vi "Modified Data File Current Mode_2.vi"(7 "Current Mode":u8[][](array[numeric]), 8 "modified error":errorcluster, 9 "modified data":path=path "C:/Users/User/Desktop/test.csv", 10 "original error":errorcluster, 11 "original data":path=path "C:/Users/User/Desktop/test.csv") -> (0 "modified data error out":errorcluster, 1 "modified data out":path, 2 "original error out":errorcluster, 3 "original data out":path)   [LabVIEW 2023]
uses:
  <vilib>/Utility/error.llb/DialogType.ctl
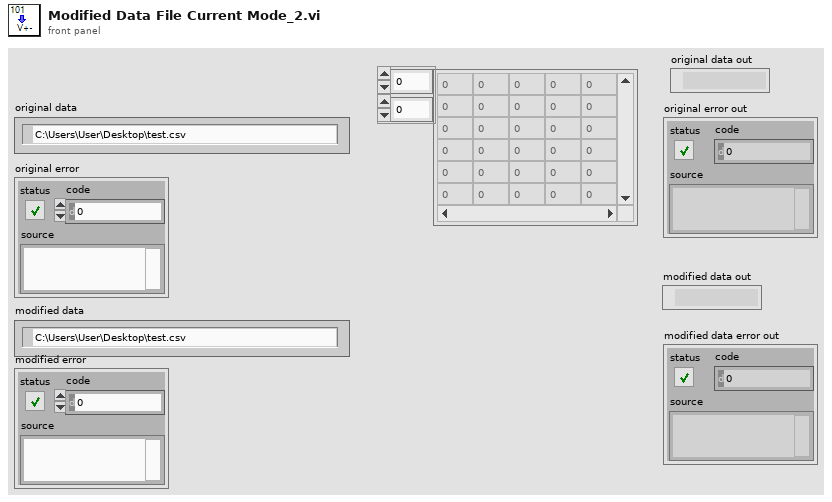
[diagram p1: front panel]
types:
  T1 = enum16{"open", "replace", "create", "open or create", "replace or create", "replace or create with confirmation"}
  T2 = typedef "DialogType.ctl" = u16
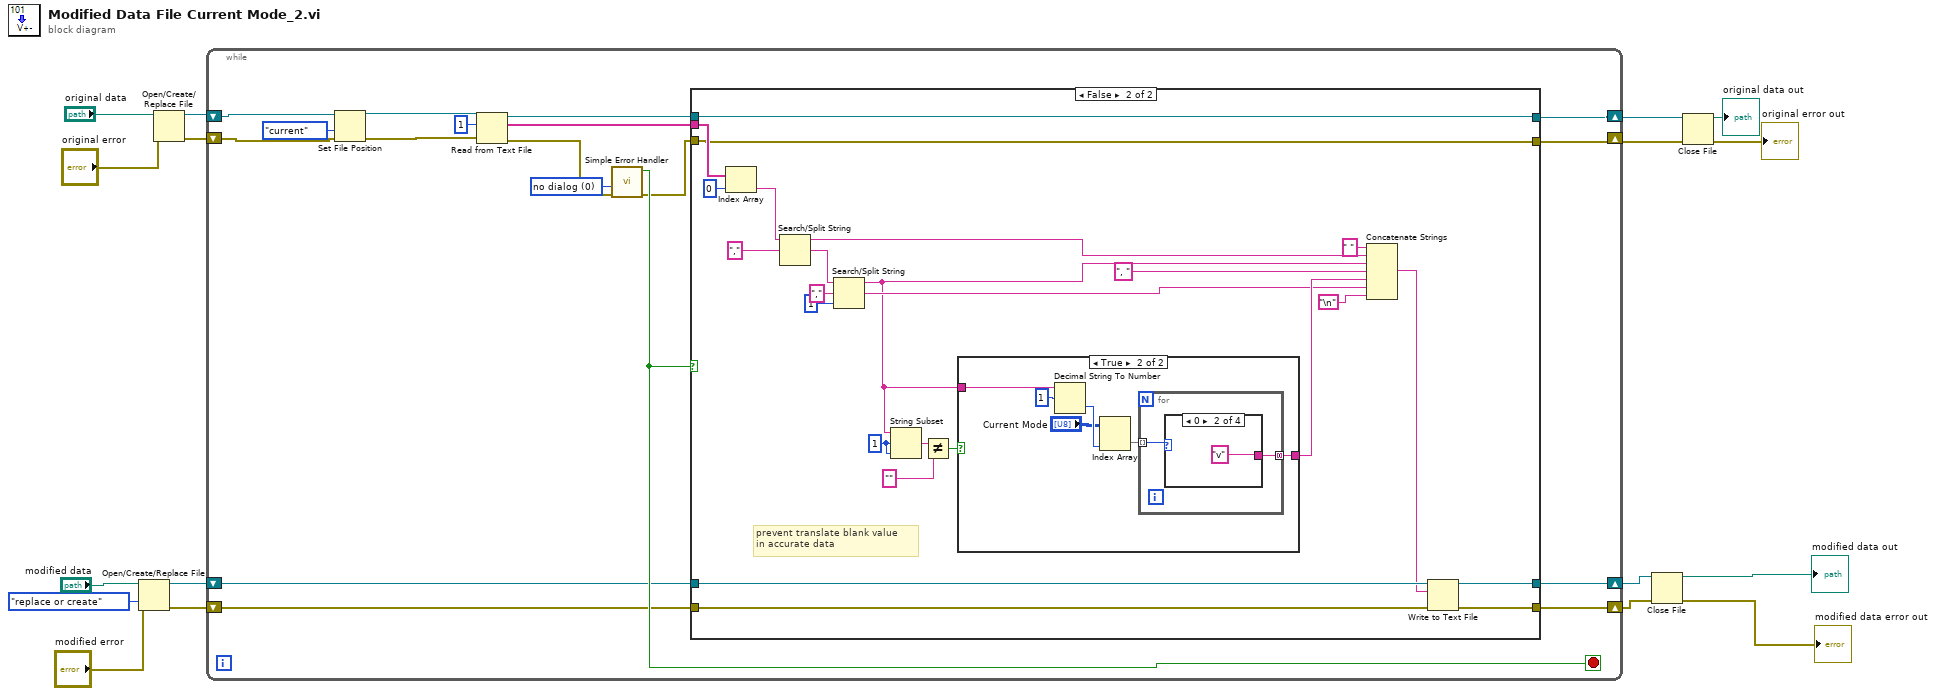
[diagram p0: block diagram]
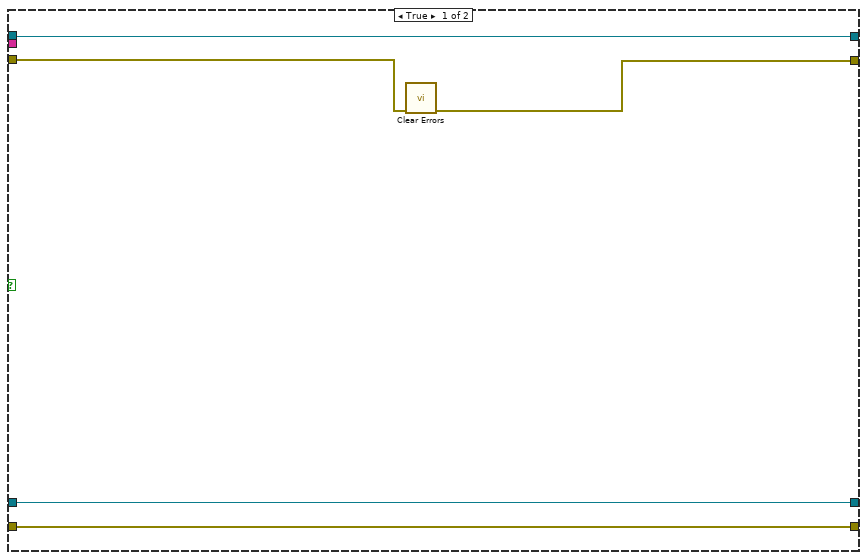
[diagram p2: hidden frame]
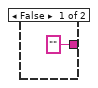
[diagram p3: hidden frame]
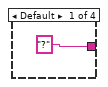
[diagram p4: hidden frame]
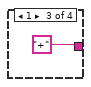
[diagram p5: hidden frame]
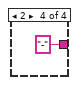
[diagram p6: hidden frame]
diagram:
  n1 = Open/Create/Replace File(file path (use dialog)="modified data", error in="modified error", operation (0:open)=T1."replace or create") -> (refnum out=w12:refnum<file>, error out=w11:errorcluster)  [unwired: 3 in, 1 out]
  n2 = Open/Create/Replace File(file path (use dialog)="original data", error in="original error") -> (refnum out=w14:refnum<file>, error out=w15:errorcluster)  [unwired: 4 in, 1 out]
  n3 = while {
    shift-right: [w27] -> w5
    shift-left: w15 -> [w34]
    shift-right: [w26] -> w16
    shift-left: w14 -> [w25]
    shift-right: [w20] -> w7
    shift-left: w12 -> [w22]
    shift-right: [w19] -> w6
    shift-left: w11 -> [w21]
    stop <- w31 stop-if-true
    w32 = T2 0 items=["no dialog", "OK message", "continue or stop message", "OK message + warnings", "continue/stop + warnings"] ("type of dialog (OK msg:1)")
    n4 = Set File Position(refnum=w25, from (0:start)=enum16{"start", "end", "current"}."current", error in=w34) -> (refnum out=w24:refnum<file>, error out=w23:errorcluster)  [unwired: 1 in]
    n5 = Read from Text File(file (use dialog)=w24, count=1, error in=w23) -> (refnum out=w29:refnum<file>, text=w30:string[], error out=w28:errorcluster)  [unwired: 1 in, 1 out]
    n6 = call <vilib>:"Simple Error Handler.vi"("type of dialog (OK msg:1)"=w32, "error in (no error)"=w28) -> ("error?"=w31:bool, "error out"=w18:errorcluster)  [unwired: 3 in, 3 out]
    n7 = case shown="False" w31 {
      tunnel: w30 -> [_ w58]
      tunnel: w29 -> [w40 w55]
      tunnel: w18 -> [w37 w54]
      tunnel: [w40 w55] -> w26
      tunnel: [w36 w54] -> w27
      tunnel: w22 -> [w39 w53]
      tunnel: w21 -> [w38 w52]
      tunnel: [w39 w51] -> w20
      tunnel: [w38 w50] -> w19
      frame True {
        n8 = call <vilib>:"Clear Errors.vi"("error in (no error)"=w37) -> ("error out"=w36:errorcluster)  [unwired: 5 in, 1 out]
      }
      frame False {
        w44 = 1 ("offset (0)")
        # "prevent translate blank value\nin accurate data"
        n9 = Index Array(array=w58, index=0) -> (element=w56:string)
        n10 = Search/Split String(string=w56, search string/char (-)=",") -> (substring before match=w64:string, match + rest of string=w63:string)  [unwired: 1 in, 1 out]
        n11 = Search/Split String(string=w63, search string/char (-)=",", offset (0)=1) -> (substring before match=w45:string, match + rest of string=w47:string)  [unwired: 1 out]
        n12 = String Subset(string=w45, offset (0)=w44, length (rest)=w44) -> (substring=w43:string)
        n13 = Not Equal?(x=w43, y="") -> (x != y?=w42:bool)
        n14 = case shown="True" w42 {
          tunnel: ["" w72] -> w65
          tunnel: w45 -> [_ w67]
          frame False {
          }
          frame True {
            n15 = Decimal String To Number(string=w67, offset=1) -> (number=w70:i32)  [unwired: 1 in, 1 out]
            n16 = Index Array(array="Current Mode", index (col)=w70) -> (element=w71:u8[])  [unwired: 1 in]
            n17 = for {
              tunnel: w71 -> [w74] mode=indexing
              tunnel: [w73] -> w72 mode=concatenating
              n18 = case shown="0" w74 {
                tunnel: ["?" "v" "+" "-"] -> w73
                frame Default {
                }
                frame 0 {
                }
                frame 1 {
                }
                frame 2 {
                }
              }
            }
          }
        }
        n19 = Concatenate Strings(" " ("string"), w64, w45, ", " ("string"), w65, w47, "\n") -> (w49:string)
        n20 = Write to Text File(file (use dialog)=w53, text=w49, error in=w52) -> (refnum out=w51:refnum<file>, error out=w50:errorcluster)  [unwired: 1 in, 1 out]
      }
    }
  }
  n21 = Close File(refnum=w7, error in=w6) -> (path=→"modified data out":path, error out=→"modified data error out":errorcluster)
  n22 = Close File(refnum=w16, error in=w5) -> (path=→"original data out":path, error out=→"original error out":errorcluster)
